vi "NavbalLabVIEW(15-5-21).vi"() -> ()   [LabVIEW 2010] (continued)
              n1265 = call "Convert from Dynamic Data7"("Dynamic Data Type"=w3197) -> ("Array"=w3196:dbl[])  [unwired: 3 in]
              n1266 = Unbundle By Name(w3189) -> ("magnitude"=w3188:dbl[])  [unwired: 2 out]
              n1267 = Array Max & Min(array=w3196) -> (max value=→"Volts":dbl)  [unwired: 3 out]
              n1268 = Array Max & Min(array=w3188) -> (max value=w3204:dbl)  [unwired: 3 out]
              "mV/in/s" <- w3204
              n1269 = case shown="True" "Save Calibration" {
                tunnel: w3204 -> [_ w3233]
                tunnel: "Calibration Channel List" -> [_ w3225]
                frame False {
                }
                frame True {
                  n1270 = local read "Boat File"() -> (w3243:path)
                  n1271 = Bundle("Calibration Channel List"=w3225, 2) -> (w3230:cluster{"Calibration Channel List":i32, i32})  [unwired: 1 in]
                  n1272 = property on="Calibration Channel List" class="MCListbox (strict)"("ActiveCell"=w3230) -> ()  [unwired: 2 in, 2 out]
                  n1273 = Add(x=w3225, y=1) -> (x+y=w3238:i32)
                  n1274 = call <vilib>:"New Report.vi"("report type"=T11."Excel", "template (empty)"=w3243) -> ("report out"=w3246:refnum<class "NI_report.lvclass">, "error out"=w3245:errorcluster)  [unwired: 12 in]
                  n1275 = Bundle(w3238, 1) -> (w3237:cluster{i32, i32})  [unwired: 1 in]
                  n1276 = Number To Fractional String(number=w3233) -> (F-format string=w3224:string)  [unwired: 3 in]
                  n1277 = call <vilib>:"Excel Get Worksheet.vi"("report in"=w3246, "worksheet index (0)"=3, "error in (no error)"=w3245) -> ("report out"=w3242:refnum<class "NI_report.lvclass">, "error out"=w3241:errorcluster)  [unwired: 11 out]
                  n1278 = property on="Calibration Channel List" class="MCListbox (strict)"() -> ("ItemNames"=w3227:string[][])  [unwired: 2 in, 2 out]
                  n1279 = Increment(x=w3225) -> (x+1=w3228:i32)
                  n1280 = call <vilib>:"Excel Easy Text.vi"("report in"=w3242, "border? (F)"=TRUE, "font"=T18 {"font name"="", "font size"=12.0, "bold"=0, "italic"=0, "underline"=0, "strike through"=0, "font color"=0}, "text"=w3224, "start (-1, -1)"=w3237, "end (-1, -1)"=w3237, "error in (no error)"=w3241) -> ("report out"=w3236:refnum<class "NI_report.lvclass">, "error out"=w3235:errorcluster)  [unwired: 4 in, 3 out]
                  n1281 = property on="Calibration Channel List" class="MCListbox (strict)"("Value"=w3228) -> ()  [unwired: 2 in, 2 out]
                  n1282 = Replace Array Subset(array=w3227, new element=w3224, index (row)=w3225, index (col)=2 ("disabled index (col)")) -> (w3223:string[][])
                  n1283 = call-dynamic "Save Report to File.vi"("report in"=w3236, "report file path"=w3243, "error in (no error)"=w3235) -> ("report out"=w3222:refnum<class "NI_report.lvclass">, "error out"=w3221:errorcluster)  [unwired: 11 in]
                  n1284 = property on="Calibration Channel List" class="MCListbox (strict)"("ItemNames"=w3223) -> ()  [unwired: 2 in, 2 out]
                  n1285 = call <vilib>:"Excel Get Last Row.vi"("report in"=w3222, "error in (no error)"=w3221) -> ("report out"=w3220:refnum<class "NI_report.lvclass">, "MS Office parameters out"=w3210:T14, "error out"=w3219:errorcluster)  [unwired: 11 in]
                  n1286 = Unbundle(w3210) -> ("position (Excel)"=w3211:cluster{"row":i32, "column":i32})  [unwired: 2 out]
                  n1287 = property on="Calibration Channel List" class="MCListbox (strict)"("CellBG"=u32 5635906) -> ()  [unwired: 2 in, 2 out]
                  n1288 = Unbundle(w3211) -> ("row"=w3212:i32)  [unwired: 1 out]
                  n1289 = Decrement(x=w3212) -> (x-1=w3214:i32)
                  n1290 = Bundle(w3214, 2) -> (w3209:cluster{i32, i32})  [unwired: 1 in]
                  n1291 = call-poly <vilib>:"Excel Get Data.vi"("report in"=w3220, "data type"=string[][] [], "start (-1, -1)"=cluster{"row":i32, "column":i32} {"row"=1, "column"=0}, "end (-1, -1)"=w3209, "error in (no error)"=w3219) -> ("data"=w3215:string[][], "error out"=w3216:errorcluster)  [unwired: 9 out]
                  n1292 = call <vilib>:"General Error Handler.vi"("error in (no error)"=w3216) -> ()  [unwired: 2 in, 13 out]
                  n1293 = local write "Sensor Info"(w3215) -> ()
                }
              }
            }
          }
        }
      }
    }
    n1294 = call <vilib>:"Value Has Changed PtByPt.vi"("input data point"="Weight Category AG") -> ("has changed"=w350:bool)  [unwired: 1 in, 1 out]
    n1295 = call <vilib>:"Value Has Changed PtByPt.vi"("input data point"="Weight Category AT") -> ("has changed"=w355:bool)  [unwired: 1 in, 1 out]
    n1296 = call <vilib>:"Value Has Changed PtByPt.vi"("input data point"="Weight Category FT") -> ("has changed"=w351:bool)  [unwired: 1 in, 1 out]
    n1297 = call <vilib>:"Value Has Changed PtByPt.vi"("input data point"="Weight Category FG") -> ("has changed"=w349:bool)  [unwired: 1 in, 1 out]
    n1298 = call <vilib>:"Value Has Changed PtByPt.vi"("input data point"="Select Side to Analyze") -> ("has changed"=w347:bool)  [unwired: 1 in, 1 out]
    n1299 = Compound Arithmetic op=OR(w347, "Refresh Button", w355, w351, w350, w349) -> (w348:bool)
    n1300 = property on="Boat File" class="Path"() -> ("Value"=w363:path)  [unwired: 2 in, 2 out]
    n1301 = property on="Tab 5" class="TabCtl (strict)"() -> ("Visible"=w364:bool)  [unwired: 2 in, 2 out]
    n1302 = case shown="\"Starboard\", Default" "Select Side to Analyze" {
      tunnel: [5 4] -> w359
      frame "Starboard", Default {
      }
      frame "Port" {
      }
    }
    n1303 = case shown="True" w364 {
      frame False {
      }
      frame True {
        # "\"12\" is the line in the excel\ndata right before the first \nchannel."
        # "PREDICTION OF MOVE"
        # "Create a list of exceptions"
        # "very long name for # of Locations/plane"
        n1304 = property on="Solution Weighting Array" class="Arr (strict)"() -> ("Index Values"=w644:u32[])  [unwired: 2 in, 2 out]
        n1305 = local read "Divisions in\nEach Plane"() -> (w643:T3)
        n1306 = local read "Holes/Division"() -> (w613:i32)
        n1307 = property on="Existing Plane Wts Port" class="Arr (strict)"() -> ("Index Values"=w635:u32[])  [unwired: 2 in, 2 out]
        n1308 = Reciprocal(x=w613) -> (1/x=w612:dbl)
        n1309 = property on="Sensor Column" class="Arr (strict)"("Index Values"=w644) -> ()  [unwired: 2 in, 2 out]
        n1310 = Array Max & Min(array=w643) -> (max value=w641:dbl)  [unwired: 3 out]
        n1311 = Multiply(x=w641, y=w613) -> (x*y=w642:dbl)
        n1312 = for {
          N: w642 -> [_]
          tunnel: [w1020] -> w640 mode=indexing
          tunnel: w612 -> [w1017]
          i -> [w1019]
          n1313 = Multiply(x=w1019, y=w1017) -> (x*y=w1018:dbl)
          n1314 = Increment(x=w1018) -> (x+1=w1020:dbl)
        }
        "Portloc" <- w640
        n1315 = property on="Existing Plane Wts Stbd" class="Arr (strict)"("Index Values"=w635) -> ()  [unwired: 2 in, 2 out]
        n1316 = property on="Portloc" class="Arr (strict)"("Index Values"=w635) -> ()  [unwired: 2 in, 2 out]
        n1317 = case shown="True" "Calc Response Coeff" {
          tunnel: [w1402 w1602] -> w600
          tunnel: [w1403 w1407] -> w646
          frame False {
            n1318 = local read "Base Complex"() -> (w1403:cdb[][])
            n1319 = local read "Response Coefficients"() -> (w1402:cdb[][])
          }
          frame True {
            w1447 = 180  # Degrees
            w1448 = 180  # Degrees
            w1481 = 0 ("disabled index (col)")
            w1532 = 0 ("disabled index (col)")
            w1561 = 0 ("disabled index (col)")
            w1537 = 180  # Degrees
            w1563 = 0 ("disabled index (col)")
            w1589 = 180  # Degrees
            w1590 = 180  # Degrees
            # "CALCULATE RESPONSE COEFFICIENTS"
            # "CALCULATE RESPONSE COEFFICIENTS"
            # "CALCULATE RESPONSE COEFFICIENTS"
            n1320 = local read "Divisions in\nEach Plane"() -> (w1446:T3)
            n1321 = local read "With/Against\nRotation"() -> (w1413:string[][])
            n1322 = local read "FT Run"() -> (w1449:sgl[][])
            n1323 = local read "AG Run"() -> (w1445:sgl[][])
            n1324 = local read "AG Wt"() -> (w1527:sgl[][])
            n1325 = local read "FG Wt"() -> (w1486:sgl[][])
            n1326 = local read "FG Run"() -> (w1444:sgl[][])
            n1327 = local read "FT Wt"() -> (w1568:sgl[][])
            n1328 = local read "AT Wt"() -> (w1558:sgl[][])
            n1329 = local read "Base Run"() -> (w1451:sgl[][])
            n1330 = local read "AT Run"() -> (w1450:sgl[][])
            n1331 = Array Size(array=w1445) -> (size(s)=w1508:i32[])
            n1332 = Index Array(array=w1508, index=1) -> (element=w1509:i32)
            n1333 = Index Array(array=w1413, index (row)=3, index (col)=0 ("disabled index (col)")) -> (element=w1417:string)
            n1334 = Index Array(array=w1413, index (row)=2, index (col)=0 ("disabled index (col)")) -> (element=w1424:string)
            n1335 = Index Array(array=w1508, index=1) -> (element=w1518:i32)
            n1336 = Array Subset "Wt Loc"(array=w1558, index (row)=0 ("index"), length (row)=1 ("length"), index (col)=1 ("index"), length (col)=1 ("index")) -> (w1465:sgl[][])
            n1337 = Array Subset "Wt Loc"(array=w1568, index (row)=1 ("index"), length (row)=1 ("length"), index (col)=1 ("index"), length (col)=1 ("index")) -> (w1463:sgl[][])
            n1338 = Array Subset "Wt Loc"(array=w1486, index (row)=3 ("index"), length (row)=1 ("length"), index (col)=1 ("index"), length (col)=1 ("index")) -> (w1461:sgl[][])
            n1339 = Array Subset "Weight"(array=w1568, index (row)=1 ("index"), length (row)=1 ("length"), index (col)=0 ("index"), length (col)=1 ("index")) -> (w1567:sgl[][])
            n1340 = Array Subset "Weight"(array=w1486, index (row)=3 ("index"), length (row)=1 ("length"), index (col)=0 ("index"), length (col)=1 ("index")) -> (w1485:sgl[][])
            n1341 = Array Size(array=w1449) -> (size(s)=w1587:i32[])
            n1342 = Array Subset "Wt Loc"(array=w1527, index (row)=2 ("index"), length (row)=1 ("length"), index (col)=1 ("index"), length (col)=1 ("index")) -> (w1462:sgl[][])
            n1343 = Array Subset "Weight"(array=w1527, index (row)=2 ("index"), length (row)=1 ("length"), index (col)=0 ("index"), length (col)=1 ("index")) -> (w1528:sgl[][])
            n1344 = Array Subset "Weight"(array=w1558, index (row)=0 ("index"), length (row)=1 ("length"), index (col)=0 ("index"), length (col)=1 ("index")) -> (w1559:sgl[][])
            n1345 = Decrement(x=w1465) -> (x-1=w1464:sgl[][])
            n1346 = Array Size(array=w1451) -> (size(s)=w1591:i32[])
            n1347 = Array Size(array=w1450) -> (size(s)=w1539:i32[])
            n1348 = Array Size(array=w1444) -> (size(s)=w1505:i32[])
            n1349 = Array Subset "Magnitude Column"(array=w1445, index (col)=0 ("index"), length (col)=w1509) -> (w1507:sgl[][])  [unwired: 2 in]
            n1350 = Array Subset "Phase Column"(array=w1445, index (col)=1 ("index"), length (col)=w1518) -> (w1515:sgl[][])  [unwired: 2 in]
            n1351 = Decrement(x=w1461) -> (x-1=w1419:sgl[][])
            n1352 = Index Array(array=w1587, index=1) -> (element=w1586:i32)
            n1353 = Decrement(x=w1463) -> (x-1=w1437:sgl[][])
            n1354 = Equal?(x="W", y=w1417) -> (x = y?=w1414:bool)
            n1355 = Equal?(x="W", y=w1424) -> (x = y?=w1422:bool)
            n1356 = Index Array(array=w1587, index=1) -> (element=w1577:i32)
            n1357 = Index Array(array=w1591, index=1) -> (element=w1592:i32)
            n1358 = Index Array(array=w1539, index=1) -> (element=w1540:i32)
            n1359 = Index Array(array=w1505, index=1) -> (element=w1504:i32)
            n1360 = Decrement(x=w1462) -> (x-1=w1428:sgl[][])
            n1361 = Index Array(array=w1591, index=1) -> (element=w1601:i32)
            n1362 = Index Array(array=w1539, index=1) -> (element=w1549:i32)
            n1363 = Index Array(array=w1505, index=1) -> (element=w1495:i32)
            n1364 = Index Array(array=w1413, index (row)=0, index (col)=0 ("disabled index (col)")) -> (element=w1441:string)
            n1365 = Divide(x=w1515, y=w1448) -> (x/y=w1514:sgl[][])
            n1366 = Index Array(array=w1413, index (row)=1, index (col)=0 ("disabled index (col)")) -> (element=w1433:string)
            n1367 = Array Subset "Magnitude Column"(array=w1449, index (col)=0 ("index"), length (col)=w1586) -> (w1588:sgl[][])  [unwired: 2 in]
            n1368 = Array Subset "Phase Column"(array=w1449, index (col)=1 ("index"), length (col)=w1577) -> (w1580:sgl[][])  [unwired: 2 in]
            n1369 = Multiply(x=w1514, y=3.141592653589793) -> (x*y=w1512:dbl[][])
            n1370 = Index Array "Choose FT number of locations"(array=w1446, index (row)=1, index (col)=0 ("disabled index (col)")) -> (element=w1435:dbl)
            n1371 = Array Subset "Magnitude Column"(array=w1451, index (col)=0 ("index"), length (col)=w1592) -> (w1466:sgl[][])  [unwired: 2 in]
            n1372 = Array Subset "Phase Column"(array=w1451, index (col)=1 ("index"), length (col)=w1601) -> (w1598:sgl[][])  [unwired: 2 in]
            n1373 = Index Array(array=w1446, index (row)=3, index (col)=0 ("disabled index (col)")) -> (element=w1421:dbl)
            n1374 = case shown="True" w1414 {
              tunnel: w1419 -> [w1637 w1645]
              tunnel: w1421 -> [w1636 w1644]
              tunnel: [w1635 w1643] -> w1420
              frame False {
                n1375 = Divide(x=w1637, y=w1636) -> (x/y=w1639:dbl[][])
                n1376 = Multiply ("Multiply.vi")(x=w1639, y=6.283185307179586) -> (x*y=w1635:dbl[][])
              }
              frame True {
                n1377 = Divide(x=w1645, y=w1644) -> (x/y=w1642:dbl[][])
                n1378 = Subtract(x=1 ("index"), y=w1642) -> (x-y=w1640:dbl[][])
                n1379 = Multiply ("Multiply.vi")(x=w1640, y=6.283185307179586) -> (x*y=w1643:dbl[][])
              }
            }
            n1380 = Array Subset "Magnitude Column"(array=w1450, index (col)=0 ("index"), length (col)=w1540) -> (w1538:sgl[][])  [unwired: 2 in]
            n1381 = Array Subset "Magnitude Column"(array=w1444, index (col)=0 ("index"), length (col)=w1504) -> (w1506:sgl[][])  [unwired: 2 in]
            n1382 = Array Subset "Phase Column"(array=w1450, index (col)=1 ("index"), length (col)=w1549) -> (w1546:sgl[][])  [unwired: 2 in]
            n1383 = Array Subset "Phase Column"(array=w1444, index (col)=1 ("index"), length (col)=w1495) -> (w1498:sgl[][])  [unwired: 2 in]
            n1384 = Index Array(array=w1446, index (row)=0, index (col)=0 ("disabled index (col)")) -> (element=w1458:dbl)
            n1385 = Index Array(array=w1446, index (row)=2, index (col)=0 ("disabled index (col)")) -> (element=w1427:dbl)
            n1386 = case shown="True" w1422 {
              tunnel: w1428 -> [w1649 w1657]
              tunnel: w1427 -> [w1648 w1656]
              tunnel: [w1647 w1655] -> w1429
              frame False {
                n1387 = Divide(x=w1649, y=w1648) -> (x/y=w1651:dbl[][])
                n1388 = Multiply ("Multiply.vi")(x=w1651, y=6.283185307179586) -> (x*y=w1647:dbl[][])
              }
              frame True {
                n1389 = Divide(x=w1657, y=w1656) -> (x/y=w1654:dbl[][])
                n1390 = Subtract(x=1 ("index"), y=w1654) -> (x-y=w1652:dbl[][])
                n1391 = Multiply ("Multiply.vi")(x=w1652, y=6.283185307179586) -> (x*y=w1655:dbl[][])
              }
            }
            n1392 = Equal?(x="W", y=w1441) -> (x = y?=w1438:bool)
            n1393 = case shown="True" w1438 {
              tunnel: w1464 -> [w1673 w1681]
              tunnel: w1458 -> [w1672 w1680]
              tunnel: [w1671 w1679] -> w1439
              frame False {
                n1394 = Divide(x=w1673, y=w1672) -> (x/y=w1675:dbl[][])
                n1395 = Multiply ("Multiply.vi")(x=w1675, y=6.283185307179586) -> (x*y=w1671:dbl[][])
              }
              frame True {
                n1396 = Divide(x=w1681, y=w1680) -> (x/y=w1678:dbl[][])
                n1397 = Subtract(x=1 ("index"), y=w1678) -> (x-y=w1676:dbl[][])
                n1398 = Multiply ("Multiply.vi")(x=w1676, y=6.283185307179586) -> (x*y=w1679:dbl[][])
              }
            }
            n1399 = Equal?(x="W", y=w1433) -> (x = y?=w1431:bool)
            n1400 = case shown="True" w1431 {
              tunnel: w1437 -> [w1661 w1669]
              tunnel: w1435 -> [w1660 w1668]
              tunnel: [w1659 w1667] -> w1436
              frame False {
                n1401 = Divide(x=w1661, y=w1660) -> (x/y=w1663:dbl[][])
                n1402 = Multiply ("Multiply.vi")(x=w1663, y=6.283185307179586) -> (x*y=w1659:dbl[][])
              }
              frame True {
                n1403 = Divide(x=w1669, y=w1668) -> (x/y=w1666:dbl[][])
                n1404 = Subtract(x=1 ("index"), y=w1666) -> (x-y=w1664:dbl[][])
                n1405 = Multiply ("Multiply.vi")(x=w1664, y=6.283185307179586) -> (x*y=w1667:dbl[][])
              }
            }
            n1406 = Divide(x=w1580, y=w1589) -> (x/y=w1581:sgl[][])
            n1407 = Polar To Complex(1:w1512, 2:w1507) -> (0:w1529:cdb[][])
            "AG Complex" <- w1529
            n1408 = Divide(x=w1598, y=w1590) -> (x/y=w1597:sgl[][])
            n1409 = Divide(x=w1546, y=w1537) -> (x/y=w1545:sgl[][])
            n1410 = Divide(x=w1498, y=w1447) -> (x/y=w1499:sgl[][])
            n1411 = Multiply(x=w1581, y=3.141592653589793) -> (x*y=w1583:dbl[][])
            n1412 = Polar To Complex ("Polar To Complex.vi")(1:w1436, 2:w1567) -> (0:w1564:cdb[][])
            n1413 = Multiply(x=w1597, y=3.141592653589793) -> (x*y=w1595:dbl[][])
            n1414 = Multiply(x=w1545, y=3.141592653589793) -> (x*y=w1543:dbl[][])
            n1415 = Multiply(x=w1499, y=3.141592653589793) -> (x*y=w1501:dbl[][])
            n1416 = Polar To Complex ("Polar To Complex.vi")(1:w1420, 2:w1485) -> (0:w1482:cdb[][])
            n1417 = Polar To Complex ("Polar To Complex.vi")(1:w1439, 2:w1559) -> (0:w1560:cdb[][])
            n1418 = Polar To Complex(1:w1583, 2:w1588) -> (0:w1566:cdb[][])
            "FT Complex" <- w1566
            n1419 = Polar To Complex(1:w1429, 2:w1528) -> (0:w1531:cdb[][])
            n1420 = Index Array(array=w1564, index (row)=w1563, index (col)=w1563) -> (element=w1562:cdb)
            n1421 = Index Array(array=w1482, index (row)=w1481, index (col)=w1481) -> (element=w1480:cdb)
            n1422 = Polar To Complex(1:w1595, 2:w1466) -> (0:w1407:cdb[][])
            n1423 = Polar To Complex(1:w1543, 2:w1538) -> (0:w1535:cdb[][])
            "AT Complex" <- w1535
            n1424 = Polar To Complex(1:w1501, 2:w1506) -> (0:w1484:cdb[][])
            "FG Complex" <- w1484
            n1425 = case shown="7" "AT Reference" {
              tunnel: w1407 -> [w1627 _ _ _ _ _ _ _]
              tunnel: [w1627 w1628 w1629 w1630 w1631 w1632 w1633 w1634] -> w1411
              frame 0, Default {
              }
              frame 1 {
                n1426 = local read "FT Complex"() -> (w1628:cdb[][])
              }
              frame 2 {
                n1427 = local read "AG Complex"() -> (w1629:cdb[][])
              }
              frame 3 {
                n1428 = local read "FG Complex"() -> (w1630:cdb[][])
              }
              frame 4 {
                n1429 = local read "Ref A"() -> (w1631:cdb[][])
              }
              frame 5 {
                n1430 = local read "Ref B"() -> (w1632:cdb[][])
              }
              frame 6 {
                n1431 = local read "Ref C"() -> (w1633:cdb[][])
              }
              frame 7 {
                n1432 = local read "Ref D"() -> (w1634:cdb[][])
              }
            }
            n1433 = Index Array(array=w1531, index (row)=w1532, index (col)=w1532) -> (element=w1533:cdb)
            n1434 = Index Array(array=w1560, index (row)=w1561, index (col)=w1561) -> (element=w1534:cdb)
            n1435 = case shown="0, Default" "AG Reference" {
              tunnel: w1407 -> [w1611 _ _ _ _ _ _ _]
              tunnel: [w1611 w1612 w1613 w1614 w1615 w1616 w1617 w1618] -> w1408
              frame 0, Default {
              }
              frame 1 {
                n1436 = local read "AT Complex"() -> (w1612:cdb[][])
              }
              frame 2 {
                n1437 = local read "FT Complex"() -> (w1613:cdb[][])
              }
              frame 3 {
                n1438 = local read "FG Complex"() -> (w1614:cdb[][])
              }
              frame 4 {
                n1439 = local read "Ref A"() -> (w1615:cdb[][])
              }
              frame 5 {
                n1440 = local read "Ref B"() -> (w1616:cdb[][])
              }
              frame 6 {
                n1441 = local read "Ref C"() -> (w1617:cdb[][])
              }
              frame 7 {
                n1442 = local read "Ref D"() -> (w1618:cdb[][])
              }
            }
            n1443 = case shown="6" "FT Reference" {
              tunnel: w1407 -> [w1619 _ _ _ _ _ _ _]
              tunnel: [w1619 w1620 w1621 w1622 w1623 w1624 w1625 w1626] -> w1409
              frame 0, Default {
              }
              frame 1 {
                n1444 = local read "AT Complex"() -> (w1620:cdb[][])
              }
              frame 2 {
                n1445 = local read "AG Complex"() -> (w1621:cdb[][])
              }
              frame 3 {
                n1446 = local read "FG Complex"() -> (w1622:cdb[][])
              }
              frame 4 {
                n1447 = local read "Ref A"() -> (w1623:cdb[][])
              }
              frame 5 {
                n1448 = local read "Ref B"() -> (w1624:cdb[][])
              }
              frame 6 {
                n1449 = local read "Ref C"() -> (w1625:cdb[][])
              }
              frame 7 {
                n1450 = local read "Ref D"() -> (w1626:cdb[][])
              }
            }
            n1451 = case shown="6" "FG Reference" {
              tunnel: w1407 -> [w1603 _ _ _ _ _ _ _]
              tunnel: [w1603 w1604 w1605 w1606 w1607 w1608 w1609 w1610] -> w1406
              frame 0, Default {
              }
              frame 1 {
                n1452 = local read "AT Complex"() -> (w1604:cdb[][])
              }
              frame 2 {
                n1453 = local read "FT Complex"() -> (w1605:cdb[][])
              }
              frame 3 {
                n1454 = local read "AG Complex"() -> (w1606:cdb[][])
              }
              frame 4 {
                n1455 = local read "Ref A"() -> (w1607:cdb[][])
              }
              frame 5 {
                n1456 = local read "Ref B"() -> (w1608:cdb[][])
              }
              frame 6 {
                n1457 = local read "Ref C"() -> (w1609:cdb[][])
              }
              frame 7 {
                n1458 = local read "Ref D"() -> (w1610:cdb[][])
              }
            }
            n1459 = Subtract(x=w1566, y=w1409) -> (x-y=w1565:cdb[][])
            n1460 = Subtract(x=w1535, y=w1411) -> (x-y=w1536:cdb[][])
            n1461 = Subtract(x=w1529, y=w1408) -> (x-y=w1530:cdb[][])
            n1462 = Subtract(x=w1484, y=w1406) -> (x-y=w1483:cdb[][])
            n1463 = Divide(x=w1565, y=w1562) -> (x/y=w1476:cdb[][])
            n1464 = Divide(x=w1536, y=w1534) -> (x/y=w1479:cdb[][])
            n1465 = Divide(x=w1530, y=w1533) -> (x/y=w1474:cdb[][])
            n1466 = Divide(x=w1483, y=w1480) -> (x/y=w1472:cdb[][])
            n1467 = Index Array "AG Port RC"(array=w1474, index (col)=0 ("disabled index (col)")) -> (element=w1469:cdb[])  [unwired: 1 in]
            n1468 = Index Array "FT Port RC"(array=w1476, index (col)=0 ("disabled index (col)")) -> (element=w1470:cdb[])  [unwired: 1 in]
            n1469 = Index Array "FG Port RC"(array=w1472, index (col)=0 ("disabled index (col)")) -> (element=w1468:cdb[])  [unwired: 1 in]
            n1470 = Index Array "AT RC"(array=w1479, index (col)=0 ("disabled index (col)")) -> (element=w1471:cdb[])  [unwired: 1 in]
            n1471 = Build Array(w1471, w1470, w1469, w1468) -> (w1467:cdb[][])
            n1472 = Transpose 2D Array(2D array=w1467) -> (transposed array=w1602:cdb[][])
          }
        }
        "Response Coefficients" <- w600
        "Base Complex" <- w646
        n1473 = property on="Boat File" class="Path"() -> ("Value"=w602:path)  [unwired: 2 in, 2 out]
        n1474 = local read "Select Side to Analyze"() -> (w611:enum32{"Starboard", "Port"})
        n1475 = case shown="True" "Empty Data Arrays" {
          frame False {
          }
          frame True {
            w1684 = dbl[][] [[0.0], [0.0], [0.0], [0.0]]
            w1683 = cdb[][] [] ("Ref B")
            w1685 = csg[] []
            w1686 = string[][] []
            w1688 = FALSE
            w1687 = i32[][] []
            n1476 = local write "Base Available"(w1688) -> ()
            n1477 = property on="Base Wt" class="Arr (strict)"("Value"=w1687) -> ()  [unwired: 2 in, 2 out]
            n1478 = property on="Base Run" class="Arr (strict)"("Value"=w1687) -> ()  [unwired: 2 in, 2 out]
            n1479 = property on="AT Wt" class="Arr (strict)"("Value"=w1687) -> ()  [unwired: 2 in, 2 out]
            n1480 = property on="AT Run" class="Arr (strict)"("Value"=w1687) -> ()  [unwired: 2 in, 2 out]
            n1481 = local write "1st Available"(w1688) -> ()
            n1482 = property on="FT Wt" class="Arr (strict)"("Value"=w1687) -> ()  [unwired: 2 in, 2 out]
            n1483 = local write "2nd Available"(w1688) -> ()
            n1484 = property on="FT Run" class="Arr (strict)"("Value"=w1687) -> ()  [unwired: 2 in, 2 out]
            n1485 = local write "3rd Available"(w1688) -> ()
            n1486 = local write "4th Available"(w1688) -> ()
            n1487 = property on="AG Wt" class="Arr (strict)"("Value"=w1687) -> ()  [unwired: 2 in, 2 out]
            n1488 = property on="AG Run" class="Arr (strict)"("Value"=w1687) -> ()  [unwired: 2 in, 2 out]
            n1489 = property on="FG Run" class="Arr (strict)"("Value"=w1687) -> ()  [unwired: 2 in, 2 out]
            n1490 = property on="FG Wt" class="Arr (strict)"("Value"=w1687) -> ()  [unwired: 2 in, 2 out]
            n1491 = property on="Response Coefficients" class="Arr (strict)"("Value"=w1687) -> ()  [unwired: 2 in, 2 out]
            n1492 = property on="AT Exceptions" class="Arr (strict)"("Value"=w1685) -> ()  [unwired: 2 in, 2 out]
            n1493 = property on="FG Exceptions" class="Arr (strict)"("Value"=w1685) -> ()  [unwired: 2 in, 2 out]
            n1494 = property on="FT Exceptions" class="Arr (strict)"("Value"=w1685) -> ()  [unwired: 2 in, 2 out]
            n1495 = property on="AG Exceptions" class="Arr (strict)"("Value"=w1685) -> ()  [unwired: 2 in, 2 out]
            n1496 = property on="Fwd Generator Balance Plane Split Options" class="MCListbox (strict)"("ItemNames"=w1686) -> ()  [unwired: 2 in, 2 out]
            n1497 = property on="Aft Turbine Balance Plane Split Options" class="MCListbox (strict)"("ItemNames"=w1686) -> ()  [unwired: 2 in, 2 out]
            n1498 = property on="Prediction Results" class="MCListbox (strict)"("ItemNames"=w1686) -> ()  [unwired: 2 in, 2 out]
            n1499 = property on="Solution Options" class="MCListbox (strict)"("ItemNames"=w1686) -> ()  [unwired: 2 in, 2 out]
            n1500 = property on="Fwd Turbine Balance Plane Split Options" class="MCListbox (strict)"("ItemNames"=w1686) -> ()  [unwired: 2 in, 2 out]
            n1501 = property on="Aft Generator Balance Plane Split Options" class="MCListbox (strict)"("ItemNames"=w1686) -> ()  [unwired: 2 in, 2 out]
            n1502 = property on="Ref C" class="Arr (strict)"("Value"=w1683) -> ()  [unwired: 2 in, 2 out]
            n1503 = property on="Ref A" class="Arr (strict)"("Value"=w1683) -> ()  [unwired: 2 in, 2 out]
            n1504 = property on="Ref B" class="Arr (strict)"("Value"=w1683) -> ()  [unwired: 2 in, 2 out]
            n1505 = property on="Ref D" class="Arr (strict)"("Value"=w1683) -> ()  [unwired: 2 in, 2 out]
            n1506 = property on="wt1" class="Arr (strict)"("Value"=w1684) -> ()  [unwired: 2 in, 2 out]
            n1507 = property on="loc1" class="Arr (strict)"("Value"=w1684) -> ()  [unwired: 2 in, 2 out]
            n1508 = property on="wt2" class="Arr (strict)"("Value"=w1684) -> ()  [unwired: 2 in, 2 out]
            n1509 = property on="loc2" class="Arr (strict)"("Value"=w1684) -> ()  [unwired: 2 in, 2 out]
          }
        }
        n1510 = case shown="\"Port\"" w611 {
          tunnel: [w824 w825] -> w609
          frame "Starboard", Default {
            n1511 = local read "#Stbd Accels"() -> (w824:i32)
          }
          frame "Port" {
            n1512 = local read "#Port Accels"() -> (w825:i32)
          }
        }
        n1513 = local read "#Corner Accels"() -> (w610:i32)
        n1514 = Add(x=w610, y=w609) -> (x+y=w608:i32)
        n1515 = Add(x=12, y=w608) -> (x+y=w606:i32)
        n1516 = Decrement(x=w606) -> (x-1=w603:i32)
        n1517 = case "Pick out Mag, Phase, and Weight locations from Excel File" shown="True" "FT Select" {
          tunnel: "Multicolumn Listbox" -> [_ w1330]
          tunnel: w602 -> [_ w1324]
          tunnel: w603 -> [_ w1313]
          frame False {
          }
          frame True {
            w1309 = string[][] []
            n1518 = local write "2nd Available"(TRUE) -> ()
            n1519 = Multiply(x=w1330, y=2) -> (x*y=w1305:i32)
            n1520 = local read "DataTab"() -> (w1323:i32)
            n1521 = Increment(x=w1305) -> (x+1=w1303:i32)
            n1522 = call <vilib>:"New Report.vi"("report type"=T11."Excel", "template (empty)"=w1324) -> ("report out"=w1331:refnum<class "NI_report.lvclass">, "error out"=w1332:errorcluster)  [unwired: 12 in]
            n1523 = Bundle("y"=12, w1303) -> (w1327:cluster{"y":i32, i32})  [unwired: 1 in]
            n1524 = call <vilib>:"Excel Get Worksheet.vi"("report in"=w1331, "worksheet index (0)"=w1323, "error in (no error)"=w1332) -> ("report out"=w1334:refnum<class "NI_report.lvclass">, "error out"=w1335:errorcluster)  [unwired: 11 out]
            n1525 = Increment(x=w1303) -> (x+1=w1304:i32)
            n1526 = Bundle(w1313, w1304) -> (w1326:cluster{i32, i32})  [unwired: 1 in]
            n1527 = call-poly <vilib>:"Excel Get Data.vi"("report in"=w1334, "data type"=w1309, "start (-1, -1)"=w1327, "end (-1, -1)"=w1326, "error in (no error)"=w1335) -> ("report out"=w1322:refnum<class "NI_report.lvclass">, "data"=w1325:string[][], "error out"=w1321:errorcluster)  [unwired: 8 out]
            n1528 = Bundle("y"=8, w1304) -> (w1317:cluster{"y":i32, i32})  [unwired: 1 in]
            n1529 = Fract/Exp String To Number(string=w1325) -> (number=→"FT Run":dbl[][])  [unwired: 3 in, 1 out]
            n1530 = Bundle("y"=5, w1303) -> (w1319:cluster{"y":i32, i32})  [unwired: 1 in]
            n1531 = call-poly <vilib>:"Excel Get Data.vi"("report in"=w1322, "data type"=w1309, "start (-1, -1)"=w1319, "end (-1, -1)"=w1317, "error in (no error)"=w1321) -> ("report out"=w1312:refnum<class "NI_report.lvclass">, "data"=w1316:string[][], "error out"=w1311:errorcluster)  [unwired: 8 out]
            n1532 = Bundle("y"=3, w1303) -> (w1308:cluster{"y":i32, i32})  [unwired: 1 in]
            n1533 = Fract/Exp String To Number(string=w1316) -> (number=→"FT Wt":dbl[][])  [unwired: 3 in, 1 out]
            n1534 = call-poly <vilib>:"Excel Get Data.vi"("report in"=w1312, "data type"=w1309, "start (-1, -1)"=w1308, "end (-1, -1)"=w1308, "error in (no error)"=w1311) -> ("error out"=w1307:errorcluster)  [unwired: 10 out]
            n1535 = call <vilib>:"General Error Handler.vi"("error in (no error)"=w1307) -> ()  [unwired: 2 in, 13 out]
          }
        }
        n1536 = case "Pick out Mag, Phase, and Weight locations from Excel File" shown="True" "Base Select" {
          tunnel: "Multicolumn Listbox" -> [_ w1396]
          tunnel: w602 -> [_ w1390]
          tunnel: w603 -> [_ w1380]
          frame False {
          }
          frame True {
            w1376 = string[][] []
            n1537 = local write "Base Available"(TRUE) -> ()
            n1538 = Multiply(x=w1396, y=2) -> (x*y=w1371:i32)
            n1539 = local read "DataTab"() -> (w1372:i32)
            n1540 = Increment(x=w1371) -> (x+1=w1369:i32)
            n1541 = call <vilib>:"New Report.vi"("report type"=T11."Excel", "template (empty)"=w1390) -> ("report out"=w1397:refnum<class "NI_report.lvclass">, "error out"=w1398:errorcluster)  [unwired: 12 in]
            n1542 = Bundle("y"=12, w1369) -> (w1393:cluster{"y":i32, i32})  [unwired: 1 in]
            n1543 = call <vilib>:"Excel Get Worksheet.vi"("report in"=w1397, "worksheet index (0)"=w1372, "error in (no error)"=w1398) -> ("report out"=w1400:refnum<class "NI_report.lvclass">, "error out"=w1401:errorcluster)  [unwired: 11 out]
            n1544 = Increment(x=w1369) -> (x+1=w1370:i32)
            n1545 = Bundle(w1380, w1370) -> (w1392:cluster{i32, i32})  [unwired: 1 in]
            n1546 = call-poly <vilib>:"Excel Get Data.vi"("report in"=w1400, "data type"=w1376, "start (-1, -1)"=w1393, "end (-1, -1)"=w1392, "error in (no error)"=w1401) -> ("report out"=w1389:refnum<class "NI_report.lvclass">, "data"=w1391:string[][], "error out"=w1388:errorcluster)  [unwired: 8 out]
            n1547 = Bundle("y"=8, w1370) -> (w1384:cluster{"y":i32, i32})  [unwired: 1 in]
            n1548 = Fract/Exp String To Number(string=w1391) -> (number=→"Base Run":dbl[][])  [unwired: 3 in, 1 out]
            n1549 = Bundle("y"=5, w1369) -> (w1386:cluster{"y":i32, i32})  [unwired: 1 in]
            n1550 = call-poly <vilib>:"Excel Get Data.vi"("report in"=w1389, "data type"=w1376, "start (-1, -1)"=w1386, "end (-1, -1)"=w1384, "error in (no error)"=w1388) -> ("report out"=w1379:refnum<class "NI_report.lvclass">, "data"=w1383:string[][], "error out"=w1378:errorcluster)  [unwired: 8 out]
            n1551 = Fract/Exp String To Number(string=w1383) -> (number=→"Base Wt":dbl[][])  [unwired: 3 in, 1 out]
            n1552 = Bundle("y"=3, w1369) -> (w1374:cluster{"y":i32, i32})  [unwired: 1 in]
            n1553 = call-poly <vilib>:"Excel Get Data.vi"("report in"=w1379, "data type"=w1376, "start (-1, -1)"=w1374, "end (-1, -1)"=w1374, "error in (no error)"=w1378) -> ("error out"=w1377:errorcluster)  [unwired: 10 out]
            n1554 = call <vilib>:"General Error Handler.vi"("error in (no error)"=w1377) -> ()  [unwired: 2 in, 13 out]
          }
        }
        n1555 = case "Pick out Mag, Phase, and Weight locations from Excel File" shown="True" "FG Select" {
          tunnel: "Multicolumn Listbox" -> [_ w1264]
          tunnel: w602 -> [_ w1258]
          tunnel: w603 -> [_ w1247]
          frame False {
          }
          frame True {
            w1242 = string[][] []
            n1556 = local write "4th Available"(TRUE) -> ()
            n1557 = Multiply(x=w1264, y=2) -> (x*y=w1239:i32)
            n1558 = local read "DataTab"() -> (w1257:i32)
            n1559 = Increment(x=w1239) -> (x+1=w1237:i32)
            n1560 = call <vilib>:"New Report.vi"("report type"=T11."Excel", "template (empty)"=w1258) -> ("report out"=w1265:refnum<class "NI_report.lvclass">, "error out"=w1266:errorcluster)  [unwired: 12 in]
            n1561 = Bundle("y"=12, w1237) -> (w1261:cluster{"y":i32, i32})  [unwired: 1 in]
            n1562 = call <vilib>:"Excel Get Worksheet.vi"("report in"=w1265, "worksheet index (0)"=w1257, "error in (no error)"=w1266) -> ("report out"=w1268:refnum<class "NI_report.lvclass">, "error out"=w1269:errorcluster)  [unwired: 11 out]
            n1563 = Increment(x=w1237) -> (x+1=w1238:i32)
            n1564 = Bundle(w1247, w1238) -> (w1260:cluster{i32, i32})  [unwired: 1 in]
            n1565 = call-poly <vilib>:"Excel Get Data.vi"("report in"=w1268, "data type"=w1242, "start (-1, -1)"=w1261, "end (-1, -1)"=w1260, "error in (no error)"=w1269) -> ("report out"=w1256:refnum<class "NI_report.lvclass">, "data"=w1259:string[][], "error out"=w1255:errorcluster)  [unwired: 8 out]
            n1566 = Bundle("y"=8, w1238) -> (w1251:cluster{"y":i32, i32})  [unwired: 1 in]
            n1567 = Bundle("y"=5, w1237) -> (w1253:cluster{"y":i32, i32})  [unwired: 1 in]
            n1568 = call-poly <vilib>:"Excel Get Data.vi"("report in"=w1256, "data type"=w1242, "start (-1, -1)"=w1253, "end (-1, -1)"=w1251, "error in (no error)"=w1255) -> ("report out"=w1243:refnum<class "NI_report.lvclass">, "data"=w1250:string[][], "error out"=w1246:errorcluster)  [unwired: 8 out]
            n1569 = Fract/Exp String To Number(string=w1259) -> (number=→"FG Run":dbl[][])  [unwired: 3 in, 1 out]
            n1570 = Bundle("y"=3, w1237) -> (w1241:cluster{"y":i32, i32})  [unwired: 1 in]
            n1571 = Fract/Exp String To Number(string=w1250) -> (number=→"FG Wt":dbl[][])  [unwired: 3 in, 1 out]
            n1572 = call-poly <vilib>:"Excel Get Data.vi"("report in"=w1243, "data type"=w1242, "start (-1, -1)"=w1241, "end (-1, -1)"=w1241, "error in (no error)"=w1246) -> ("error out"=w1245:errorcluster)  [unwired: 10 out]
            n1573 = call <vilib>:"General Error Handler.vi"("error in (no error)"=w1245) -> ()  [unwired: 2 in, 13 out]
          }
        }
        n1574 = case "Pick out Mag, Phase, and Weight locations from Excel File" shown="True" "AT Select" {
          tunnel: "Multicolumn Listbox" -> [_ w1363]
          tunnel: w602 -> [_ w1357]
          tunnel: w603 -> [_ w1346]
          frame False {
          }
          frame True {
            w1342 = string[][] []
            n1575 = local write "1st Available"(TRUE) -> ()
            n1576 = Multiply(x=w1363, y=2) -> (x*y=w1338:i32)
            n1577 = local read "DataTab"() -> (w1356:i32)
            n1578 = Increment(x=w1338) -> (x+1=w1336:i32)
            n1579 = call <vilib>:"New Report.vi"("report type"=T11."Excel", "template (empty)"=w1357) -> ("report out"=w1364:refnum<class "NI_report.lvclass">, "error out"=w1365:errorcluster)  [unwired: 12 in]
            n1580 = Bundle("y"=12, w1336) -> (w1360:cluster{"y":i32, i32})  [unwired: 1 in]
            n1581 = call <vilib>:"Excel Get Worksheet.vi"("report in"=w1364, "worksheet index (0)"=w1356, "error in (no error)"=w1365) -> ("report out"=w1367:refnum<class "NI_report.lvclass">, "error out"=w1368:errorcluster)  [unwired: 11 out]
            n1582 = Increment(x=w1336) -> (x+1=w1337:i32)
            n1583 = Bundle(w1346, w1337) -> (w1359:cluster{i32, i32})  [unwired: 1 in]
            n1584 = call-poly <vilib>:"Excel Get Data.vi"("report in"=w1367, "data type"=w1342, "start (-1, -1)"=w1360, "end (-1, -1)"=w1359, "error in (no error)"=w1368) -> ("report out"=w1355:refnum<class "NI_report.lvclass">, "data"=w1358:string[][], "error out"=w1354:errorcluster)  [unwired: 8 out]
            n1585 = Bundle("y"=8, w1337) -> (w1350:cluster{"y":i32, i32})  [unwired: 1 in]
            n1586 = Bundle("y"=5, w1336) -> (w1352:cluster{"y":i32, i32})  [unwired: 1 in]
            n1587 = call-poly <vilib>:"Excel Get Data.vi"("report in"=w1355, "data type"=w1342, "start (-1, -1)"=w1352, "end (-1, -1)"=w1350, "error in (no error)"=w1354) -> ("report out"=w1344:refnum<class "NI_report.lvclass">, "data"=w1349:string[][], "error out"=w1345:errorcluster)  [unwired: 8 out]
            n1588 = Fract/Exp String To Number(string=w1358) -> (number=→"AT Run":dbl[][])  [unwired: 3 in, 1 out]
            n1589 = Fract/Exp String To Number(string=w1349) -> (number=→"AT Wt":dbl[][])  [unwired: 3 in, 1 out]
            n1590 = Bundle("y"=3, w1336) -> (w1341:cluster{"y":i32, i32})  [unwired: 1 in]
            n1591 = call-poly <vilib>:"Excel Get Data.vi"("report in"=w1344, "data type"=w1342, "start (-1, -1)"=w1341, "end (-1, -1)"=w1341, "error in (no error)"=w1345) -> ("error out"=w1340:errorcluster)  [unwired: 10 out]
            n1592 = call <vilib>:"General Error Handler.vi"("error in (no error)"=w1340) -> ()  [unwired: 2 in, 13 out]
          }
        }
        n1593 = case "Pick out Mag, Phase, and Weight locations from Excel File" shown="True" "AG Select" {
          tunnel: "Multicolumn Listbox" -> [_ w1297]
          tunnel: w602 -> [_ w1291]
          tunnel: w603 -> [_ w1280]
          frame False {
          }
          frame True {
            w1278 = string[][] []
            n1594 = local write "3rd Available"(TRUE) -> ()
            n1595 = Multiply(x=w1297, y=2) -> (x*y=w1272:i32)
            n1596 = local read "DataTab"() -> (w1290:i32)
            n1597 = Increment(x=w1272) -> (x+1=w1270:i32)
            n1598 = call <vilib>:"New Report.vi"("report type"=T11."Excel", "template (empty)"=w1291) -> ("report out"=w1298:refnum<class "NI_report.lvclass">, "error out"=w1299:errorcluster)  [unwired: 12 in]
            n1599 = Bundle("y"=12, w1270) -> (w1294:cluster{"y":i32, i32})  [unwired: 1 in]
            n1600 = call <vilib>:"Excel Get Worksheet.vi"("report in"=w1298, "worksheet index (0)"=w1290, "error in (no error)"=w1299) -> ("report out"=w1301:refnum<class "NI_report.lvclass">, "error out"=w1302:errorcluster)  [unwired: 11 out]
            n1601 = Increment(x=w1270) -> (x+1=w1271:i32)
            n1602 = Bundle(w1280, w1271) -> (w1293:cluster{i32, i32})  [unwired: 1 in]
            n1603 = call-poly <vilib>:"Excel Get Data.vi"("report in"=w1301, "data type"=w1278, "start (-1, -1)"=w1294, "end (-1, -1)"=w1293, "error in (no error)"=w1302) -> ("report out"=w1289:refnum<class "NI_report.lvclass">, "data"=w1292:string[][], "error out"=w1288:errorcluster)  [unwired: 8 out]
            n1604 = Bundle("y"=8, w1271) -> (w1284:cluster{"y":i32, i32})  [unwired: 1 in]
            n1605 = Bundle("y"=5, w1270) -> (w1286:cluster{"y":i32, i32})  [unwired: 1 in]
            n1606 = call-poly <vilib>:"Excel Get Data.vi"("report in"=w1289, "data type"=w1278, "start (-1, -1)"=w1286, "end (-1, -1)"=w1284, "error in (no error)"=w1288) -> ("report out"=w1275:refnum<class "NI_report.lvclass">, "data"=w1283:string[][], "error out"=w1279:errorcluster)  [unwired: 8 out]
            n1607 = Fract/Exp String To Number(string=w1292) -> (number=→"AG Run":dbl[][])  [unwired: 3 in, 1 out]
            n1608 = Fract/Exp String To Number(string=w1283) -> (number=→"AG Wt":dbl[][])  [unwired: 3 in, 1 out]
            n1609 = Bundle("y"=3, w1270) -> (w1276:cluster{"y":i32, i32})  [unwired: 1 in]
            n1610 = call-poly <vilib>:"Excel Get Data.vi"("report in"=w1275, "data type"=w1278, "start (-1, -1)"=w1276, "end (-1, -1)"=w1276, "error in (no error)"=w1279) -> ("error out"=w1274:errorcluster)  [unwired: 10 out]
            n1611 = call <vilib>:"General Error Handler.vi"("error in (no error)"=w1274) -> ()  [unwired: 2 in, 13 out]
          }
        }
        n1612 = local read "Divisions in\nEach Plane"() -> (w605:T3)
        n1613 = case shown="True" "Calculate 2 wt" {
          tunnel: w605 -> [_ w991]
          frame False {
          }
          frame True {
            n1614 = Decrement(x="loc1") -> (x-1=w1007:T3)
            n1615 = Decrement(x="loc2") -> (x-1=w1001:T3)
            n1616 = call-poly <vilib>:"Matrix To Array.vi"("Real Matrix"=w991) -> ("Real 2D Array"=w989:dbl[][])
            n1617 = Divide(x=w1001, y=w989) -> (x/y=w1002:T3)
            n1618 = Divide(x=w1007, y=w989) -> (x/y=w1006:T3)
            n1619 = call-poly <vilib>:"Multiply.vi"("Real Scalar c"=6.283185307179586, "Real Matrix A"=w1002) -> ("A * c"=w999:T3)
            n1620 = call-poly <vilib>:"Multiply.vi"("Real Scalar c"=6.283185307179586, "Real Matrix A"=w1006) -> ("A * c"=w1004:T3)
            n1621 = call-poly <vilib>:"Polar To Complex.vi"("Argument Q"=w999, "Modulus r"="wt2") -> ("Complex Matrix r*e^iQ"=w996:T15)
            n1622 = call-poly <vilib>:"Polar To Complex.vi"("Argument Q"=w1004, "Modulus r"="wt1") -> ("Complex Matrix r*e^iQ"=w997:T15)
            n1623 = call-poly <vilib>:"Add.vi"("Complex Matrix B"=w996, "Complex Matrix A"=w997) -> ("A + B"=w995:T15)
            n1624 = call-poly <vilib>:"Complex To Polar.vi"("Complex Matrix r*e^iQ"=w995) -> ("Modulus r"=w994:T3, "Argument Q"=w988:T3)
            n1625 = for {
              tunnel: w988 -> [w1011] mode=indexing
              tunnel: [w1010] -> w987 mode=indexing
              n1626 = for {
                tunnel: w1011 -> [w1013] mode=indexing
                tunnel: [w1012] -> w1010 mode=indexing
                n1627 = Less Than 0?(x=w1013) -> (x < 0?=w1014:bool)
                n1628 = Add ("Add.vi")(x=w1013, y=6.283185307179586) -> (x+y=w1016:dbl)
                n1629 = Select(t=w1016, s=w1014, f=w1013) -> (s? t:f=w1012:dbl)
              }
            }
            n1630 = local write "Correction Mag"(w994) -> ()
            n1631 = Divide(x=w987, y=6.283185307179586) -> (x/y=w986:dbl[][])
            n1632 = Multiply(x=w989, y=w986) -> (x*y=w990:dbl[][])
            n1633 = Increment(x=w990) -> (x+1=w992:dbl[][])
            n1634 = local write "Correction Loc"(w992) -> ()
          }
        }
        n1635 = case "Pick out Mag, Phase, and Weight locations from Excel File" shown="True" "Ref C Select" {
          tunnel: "Multicolumn Listbox" -> [_ w892]
          tunnel: w602 -> [_ w887]
          tunnel: w603 -> [_ w879]
          frame False {
          }
          frame True {
            w856 = 180  # Degrees
            w875 = string[][] []
            n1636 = Multiply(x=w892, y=2) -> (x*y=w871:i32)
            n1637 = local read "DataTab"() -> (w886:i32)
            n1638 = Increment(x=w871) -> (x+1=w869:i32)
            n1639 = call <vilib>:"New Report.vi"("report type"=T11."Excel", "template (empty)"=w887) -> ("report out"=w893:refnum<class "NI_report.lvclass">, "error out"=w894:errorcluster)  [unwired: 12 in]
            n1640 = Bundle("y"=12, w869) -> (w890:cluster{"y":i32, i32})  [unwired: 1 in]
            n1641 = call <vilib>:"Excel Get Worksheet.vi"("report in"=w893, "worksheet index (0)"=w886, "error in (no error)"=w894) -> ("report out"=w896:refnum<class "NI_report.lvclass">, "error out"=w897:errorcluster)  [unwired: 11 out]
            n1642 = Increment(x=w869) -> (x+1=w870:i32)
            n1643 = Bundle(w879, w870) -> (w889:cluster{i32, i32})  [unwired: 1 in]
            n1644 = call-poly <vilib>:"Excel Get Data.vi"("report in"=w896, "data type"=w875, "start (-1, -1)"=w890, "end (-1, -1)"=w889, "error in (no error)"=w897) -> ("report out"=w885:refnum<class "NI_report.lvclass">, "data"=w888:string[][], "error out"=w884:errorcluster)  [unwired: 8 out]
            n1645 = Bundle("y"=8, w870) -> (w880:cluster{"y":i32, i32})  [unwired: 1 in]
            n1646 = Bundle("y"=5, w869) -> (w882:cluster{"y":i32, i32})  [unwired: 1 in]
            n1647 = call-poly <vilib>:"Excel Get Data.vi"("report in"=w885, "data type"=w875, "start (-1, -1)"=w882, "end (-1, -1)"=w880, "error in (no error)"=w884) -> ("report out"=w877:refnum<class "NI_report.lvclass">, "error out"=w878:errorcluster)  [unwired: 9 out]
            n1648 = Fract/Exp String To Number(string=w888) -> (number=w855:dbl[][])  [unwired: 3 in, 1 out]
            n1649 = Bundle("y"=3, w869) -> (w874:cluster{"y":i32, i32})  [unwired: 1 in]
            n1650 = call-poly <vilib>:"Excel Get Data.vi"("report in"=w877, "data type"=w875, "start (-1, -1)"=w874, "end (-1, -1)"=w874, "error in (no error)"=w878) -> ("error out"=w873:errorcluster)  [unwired: 10 out]
            n1651 = call <vilib>:"General Error Handler.vi"("error in (no error)"=w873) -> ()  [unwired: 2 in, 13 out]
            n1652 = Array Size(array=w855) -> (size(s)=w867:i32[])
            n1653 = Index Array(array=w867, index=1) -> (element=w866:i32)
            n1654 = Index Array(array=w867, index=1) -> (element=w857:i32)
            n1655 = Array Subset "Magnitude Column"(array=w855, index (col)=0 ("index"), length (col)=w866) -> (w868:dbl[][])  [unwired: 2 in]
            n1656 = Array Subset "Phase Column"(array=w855, index (col)=1 ("index"), length (col)=w857) -> (w860:dbl[][])  [unwired: 2 in]
            n1657 = Divide(x=w860, y=w856) -> (x/y=w861:dbl[][])
            n1658 = Multiply(x=w861, y=3.141592653589793) -> (x*y=w863:dbl[][])
            n1659 = Polar To Complex(1:w863, 2:w868) -> (0:→"Ref C":cdb[][])
          }
        }
        n1660 = case "Pick out Mag, Phase, and Weight locations from Excel File" shown="True" "Ref D Select" {
          tunnel: "Multicolumn Listbox" -> [_ w696]
          tunnel: w602 -> [_ w691]
          tunnel: w603 -> [_ w683]
          frame False {
          }
          frame True {
            w660 = 180  # Degrees
            w679 = string[][] []
            n1661 = Multiply(x=w696, y=2) -> (x*y=w675:i32)
            n1662 = local read "DataTab"() -> (w690:i32)
            n1663 = Increment(x=w675) -> (x+1=w673:i32)
            n1664 = call <vilib>:"New Report.vi"("report type"=T11."Excel", "template (empty)"=w691) -> ("report out"=w697:refnum<class "NI_report.lvclass">, "error out"=w698:errorcluster)  [unwired: 12 in]
            n1665 = Bundle("y"=12, w673) -> (w694:cluster{"y":i32, i32})  [unwired: 1 in]
            n1666 = call <vilib>:"Excel Get Worksheet.vi"("report in"=w697, "worksheet index (0)"=w690, "error in (no error)"=w698) -> ("report out"=w700:refnum<class "NI_report.lvclass">, "error out"=w701:errorcluster)  [unwired: 11 out]
            n1667 = Increment(x=w673) -> (x+1=w674:i32)
            n1668 = Bundle(w683, w674) -> (w693:cluster{i32, i32})  [unwired: 1 in]
            n1669 = call-poly <vilib>:"Excel Get Data.vi"("report in"=w700, "data type"=w679, "start (-1, -1)"=w694, "end (-1, -1)"=w693, "error in (no error)"=w701) -> ("report out"=w689:refnum<class "NI_report.lvclass">, "data"=w692:string[][], "error out"=w688:errorcluster)  [unwired: 8 out]
            n1670 = Bundle("y"=8, w674) -> (w684:cluster{"y":i32, i32})  [unwired: 1 in]
            n1671 = Bundle("y"=5, w673) -> (w686:cluster{"y":i32, i32})  [unwired: 1 in]
            n1672 = call-poly <vilib>:"Excel Get Data.vi"("report in"=w689, "data type"=w679, "start (-1, -1)"=w686, "end (-1, -1)"=w684, "error in (no error)"=w688) -> ("report out"=w681:refnum<class "NI_report.lvclass">, "error out"=w682:errorcluster)  [unwired: 9 out]
            n1673 = Fract/Exp String To Number(string=w692) -> (number=w659:dbl[][])  [unwired: 3 in, 1 out]
            n1674 = Bundle("y"=3, w673) -> (w678:cluster{"y":i32, i32})  [unwired: 1 in]
            n1675 = call-poly <vilib>:"Excel Get Data.vi"("report in"=w681, "data type"=w679, "start (-1, -1)"=w678, "end (-1, -1)"=w678, "error in (no error)"=w682) -> ("error out"=w677:errorcluster)  [unwired: 10 out]
            n1676 = call <vilib>:"General Error Handler.vi"("error in (no error)"=w677) -> ()  [unwired: 2 in, 13 out]
            n1677 = Array Size(array=w659) -> (size(s)=w671:i32[])
            n1678 = Index Array(array=w671, index=1) -> (element=w670:i32)
            n1679 = Index Array(array=w671, index=1) -> (element=w661:i32)
            n1680 = Array Subset "Magnitude Column"(array=w659, index (col)=0 ("index"), length (col)=w670) -> (w672:dbl[][])  [unwired: 2 in]
            n1681 = Array Subset "Phase Column"(array=w659, index (col)=1 ("index"), length (col)=w661) -> (w664:dbl[][])  [unwired: 2 in]
            n1682 = Divide(x=w664, y=w660) -> (x/y=w665:dbl[][])
            n1683 = Multiply(x=w665, y=3.141592653589793) -> (x*y=w667:dbl[][])
            n1684 = Polar To Complex(1:w667, 2:w672) -> (0:→"Ref D":cdb[][])
          }
        }
        n1685 = case "Choose an alternative Reference A for" shown="True" "Ref A Select" {
          tunnel: "Multicolumn Listbox" -> [_ w980]
          tunnel: w602 -> [_ w974]
          tunnel: w603 -> [_ w966]
          frame False {
          }
          frame True {
            w943 = 180  # Degrees
            w962 = string[][] []
            n1686 = Multiply(x=w980, y=2) -> (x*y=w959:i32)
            n1687 = local read "DataTab"() -> (w973:i32)
            n1688 = Increment(x=w959) -> (x+1=w957:i32)
            n1689 = call <vilib>:"New Report.vi"("report type"=T11."Excel", "template (empty)"=w974) -> ("report out"=w981:refnum<class "NI_report.lvclass">, "error out"=w982:errorcluster)  [unwired: 12 in]
            n1690 = Bundle("y"=12, w957) -> (w977:cluster{"y":i32, i32})  [unwired: 1 in]
            n1691 = call <vilib>:"Excel Get Worksheet.vi"("report in"=w981, "worksheet index (0)"=w973, "error in (no error)"=w982) -> ("report out"=w984:refnum<class "NI_report.lvclass">, "error out"=w985:errorcluster)  [unwired: 11 out]
            n1692 = Increment(x=w957) -> (x+1=w958:i32)
            n1693 = Bundle(w966, w958) -> (w976:cluster{i32, i32})  [unwired: 1 in]
            n1694 = call-poly <vilib>:"Excel Get Data.vi"("report in"=w984, "data type"=w962, "start (-1, -1)"=w977, "end (-1, -1)"=w976, "error in (no error)"=w985) -> ("report out"=w972:refnum<class "NI_report.lvclass">, "data"=w975:string[][], "error out"=w971:errorcluster)  [unwired: 8 out]
            n1695 = Bundle("y"=8, w958) -> (w967:cluster{"y":i32, i32})  [unwired: 1 in]
            n1696 = Bundle("y"=5, w957) -> (w969:cluster{"y":i32, i32})  [unwired: 1 in]
            n1697 = call-poly <vilib>:"Excel Get Data.vi"("report in"=w972, "data type"=w962, "start (-1, -1)"=w969, "end (-1, -1)"=w967, "error in (no error)"=w971) -> ("report out"=w964:refnum<class "NI_report.lvclass">, "error out"=w965:errorcluster)  [unwired: 9 out]
            n1698 = Fract/Exp String To Number(string=w975) -> (number=w944:dbl[][])  [unwired: 3 in, 1 out]
            n1699 = Bundle("y"=3, w957) -> (w961:cluster{"y":i32, i32})  [unwired: 1 in]
            n1700 = call-poly <vilib>:"Excel Get Data.vi"("report in"=w964, "data type"=w962, "start (-1, -1)"=w961, "end (-1, -1)"=w961, "error in (no error)"=w965) -> ("error out"=w960:errorcluster)  [unwired: 10 out]
            n1701 = call <vilib>:"General Error Handler.vi"("error in (no error)"=w960) -> ()  [unwired: 2 in, 13 out]
            n1702 = Array Size(array=w944) -> (size(s)=w955:i32[])
            n1703 = Index Array(array=w955, index=1) -> (element=w954:i32)
            n1704 = Index Array(array=w955, index=1) -> (element=w945:i32)
            n1705 = Array Subset "Magnitude Column"(array=w944, index (col)=0 ("index"), length (col)=w954) -> (w956:dbl[][])  [unwired: 2 in]
            n1706 = Array Subset "Phase Column"(array=w944, index (col)=1 ("index"), length (col)=w945) -> (w948:dbl[][])  [unwired: 2 in]
            n1707 = Divide(x=w948, y=w943) -> (x/y=w949:dbl[][])
            n1708 = Multiply(x=w949, y=3.141592653589793) -> (x*y=w951:dbl[][])
            n1709 = Polar To Complex(1:w951, 2:w956) -> (0:→"Ref A":cdb[][])
          }
        }
        n1710 = case "Pick out Mag, Phase, and Weight locations from Excel File" shown="True" "Ref B Select" {
          tunnel: "Multicolumn Listbox" -> [_ w936]
          tunnel: w602 -> [_ w930]
          tunnel: w603 -> [_ w922]
          frame False {
          }
          frame True {
            w912 = 180  # Degrees
            w918 = string[][] []
            n1711 = Multiply(x=w936, y=2) -> (x*y=w915:i32)
            n1712 = local read "DataTab"() -> (w929:i32)
            n1713 = Increment(x=w915) -> (x+1=w913:i32)
            n1714 = call <vilib>:"New Report.vi"("report type"=T11."Excel", "template (empty)"=w930) -> ("report out"=w937:refnum<class "NI_report.lvclass">, "error out"=w938:errorcluster)  [unwired: 12 in]
            n1715 = Bundle("y"=12, w913) -> (w933:cluster{"y":i32, i32})  [unwired: 1 in]
            n1716 = call <vilib>:"Excel Get Worksheet.vi"("report in"=w937, "worksheet index (0)"=w929, "error in (no error)"=w938) -> ("report out"=w940:refnum<class "NI_report.lvclass">, "error out"=w941:errorcluster)  [unwired: 11 out]
            n1717 = Increment(x=w913) -> (x+1=w914:i32)
            n1718 = Bundle(w922, w914) -> (w932:cluster{i32, i32})  [unwired: 1 in]
            n1719 = call-poly <vilib>:"Excel Get Data.vi"("report in"=w940, "data type"=w918, "start (-1, -1)"=w933, "end (-1, -1)"=w932, "error in (no error)"=w941) -> ("report out"=w928:refnum<class "NI_report.lvclass">, "data"=w931:string[][], "error out"=w927:errorcluster)  [unwired: 8 out]
            n1720 = Bundle("y"=8, w914) -> (w923:cluster{"y":i32, i32})  [unwired: 1 in]
            n1721 = Bundle("y"=5, w913) -> (w925:cluster{"y":i32, i32})  [unwired: 1 in]
            n1722 = call-poly <vilib>:"Excel Get Data.vi"("report in"=w928, "data type"=w918, "start (-1, -1)"=w925, "end (-1, -1)"=w923, "error in (no error)"=w927) -> ("report out"=w920:refnum<class "NI_report.lvclass">, "error out"=w921:errorcluster)  [unwired: 9 out]
            n1723 = Fract/Exp String To Number(string=w931) -> (number=w899:dbl[][])  [unwired: 3 in, 1 out]
            n1724 = Bundle("y"=3, w913) -> (w917:cluster{"y":i32, i32})  [unwired: 1 in]
            n1725 = call-poly <vilib>:"Excel Get Data.vi"("report in"=w920, "data type"=w918, "start (-1, -1)"=w917, "end (-1, -1)"=w917, "error in (no error)"=w921) -> ("error out"=w916:errorcluster)  [unwired: 10 out]
            n1726 = call <vilib>:"General Error Handler.vi"("error in (no error)"=w916) -> ()  [unwired: 2 in, 13 out]
            n1727 = Array Size(array=w899) -> (size(s)=w901:i32[])
            n1728 = Index Array(array=w901, index=1) -> (element=w902:i32)
            n1729 = Index Array(array=w901, index=1) -> (element=w911:i32)
            n1730 = Array Subset "Magnitude Column"(array=w899, index (col)=0 ("index"), length (col)=w902) -> (w900:dbl[][])  [unwired: 2 in]
            n1731 = Array Subset "Phase Column"(array=w899, index (col)=1 ("index"), length (col)=w911) -> (w908:dbl[][])  [unwired: 2 in]
            n1732 = Divide(x=w908, y=w912) -> (x/y=w907:dbl[][])
            n1733 = Multiply(x=w907, y=3.141592653589793) -> (x*y=w905:dbl[][])
            n1734 = Polar To Complex(1:w905, 2:w900) -> (0:→"Ref B":cdb[][])
          }
        }
        n1735 = flat-sequence {
          tunnel: w605 -> [w702]
          frame #0 {
            n1736 = Index Array(array=w702, index (col)=0 ("disabled index (col)")) -> (element=w708:dbl[])  [unwired: 1 in]
            n1737 = local read "With/Against\nRotation"() -> (w713:string[][])
            n1738 = Index Array(array="Correction Loc", index (col)=0 ("disabled index (col)")) -> (element=w705:dbl[])  [unwired: 1 in]
            n1739 = Array Size(array=w705) -> (size(s)=w706:i32)
            n1740 = Index Array(array=w713, index (col)=0 ("disabled index (col)")) -> (element=w715:string[])  [unwired: 1 in]
            n1741 = for {
              N: w706 -> [_]
              tunnel: w705 -> [w721] mode=indexing
              tunnel: w708 -> [w720] mode=indexing
              tunnel: [w719] -> w709 mode=indexing
              tunnel: w715 -> [w718] mode=indexing
              n1742 = Equal?(x=w718, y="W") -> (x = y?=w716:bool)
              n1743 = case shown="True" w716 {
                tunnel: w721 -> [w727 w735]
                tunnel: w720 -> [w724 w732]
                tunnel: [w722 w730] -> w719
                frame False {
                  n1744 = Decrement(x=w727) -> (x-1=w726:dbl)
                  n1745 = Divide(x=360.0, y=w724) -> (x/y=w723:dbl)
                  n1746 = Multiply(x=w723, y=w726) -> (x*y=w722:dbl)
                }
                frame True {
                  n1747 = Decrement(x=w735) -> (x-1=w734:dbl)
                  n1748 = Divide(x=360.0, y=w732) -> (x/y=w731:dbl)
                  n1749 = Multiply(x=w731, y=w734) -> (x*y=w729:dbl)
                  n1750 = Subtract(x=360.0, y=w729) -> (x-y=w730:dbl)
                }
              }
            }
            n1751 = Reshape Array(w709, 4 ("dimension size"), 1 ("dimension size")) -> (w712:dbl[][])
            n1752 = local write "Correction Phase"(w712) -> ()
          }
          frame #1 {
            w782 = i16 3 ("precision (6)")
            # "Add Correction \nto Baseline Vibes"
            # "Calc Effect of Masses"
            n1753 = local read "Startpt Complex"() -> (w743:cdb[][])
            n1754 = Divide(x="Correction Phase", y=180) -> (x/y=w807:T3)
            n1755 = Complex To Polar(r * e^(i*theta)=w743) -> (r=w795:dbl[][], theta=w796:dbl[][])
            n1756 = call-poly <vilib>:"Multiply.vi"("Real Scalar c"=3.141592653589793, "Real Matrix A"=w807) -> ("A * c"=w805:T3)
            n1757 = Divide(x=w796, y=3.141592653589793) -> (x/y=w792:dbl[][])
